vi "AlazarSetTriggerOperation.vi"(0 "Handle":u64, 1 "Trigger Operation":u32(ring) items=["J", "K", "J OR K", "J AND K", "J XOR K", "J AND NOT K", "NOT J AND K"], 5 "error in (no error)":errorcluster, 6 "Trigger Engine 1":u32(ring) items=["J", "K"], 7 "Trigger Engine 2":u32(ring)=1 items=["J", "K"], 8 "Source 1":u32(ring) items=["A", "B", "External", "Disable", "C", "D"], 9 "Source 2":u32(ring)=3 items=["A", "B", "External", "Disable", "C", "D"], 10 "Slope 1":u32(ring)=1 items=["Positive"=1, "Negative"=2], 11 "Slope 2":u32(ring)=1 items=["Positive"=1, "Negative"=2], 12 "Level 1":u32, 13 "Level 2":u32) -> (14 "Handle":u64, 18 "Return Code":u32, 19 "error out":errorcluster)   [LabVIEW 2018]
doc: "Configure the trigger system."
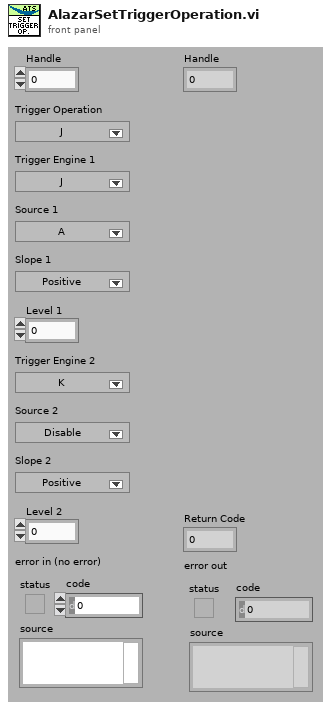
[diagram p1: front panel]
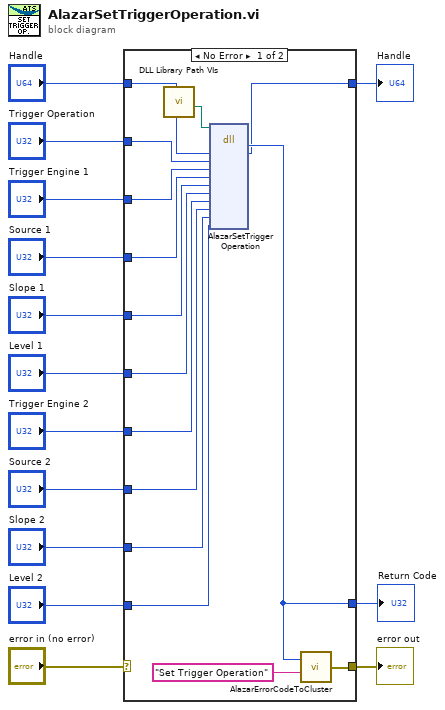
[diagram p0: block diagram]
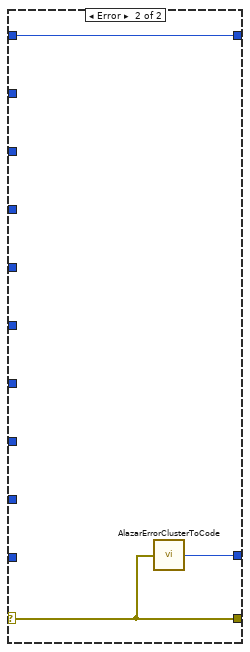
[diagram p2: hidden frame]
diagram:
  n1 = case shown="No Error" "error in (no error)" {
    selector: "error in (no error)" -> [_ w32]
    tunnel: [w26 w32] -> w13
    tunnel: [w28 w31] -> w12
    tunnel: "Handle" -> [w29 w30]
    tunnel: [w25 w30] -> w10
    tunnel: "Trigger Operation" -> [w24 _]
    tunnel: "Trigger Engine 1" -> [w23 _]
    tunnel: "Source 1" -> [w22 _]
    tunnel: "Slope 1" -> [w21 _]
    tunnel: "Level 1" -> [w20 _]
    tunnel: "Trigger Engine 2" -> [w19 _]
    tunnel: "Source 2" -> [w18 _]
    tunnel: "Slope 2" -> [w17 _]
    tunnel: "Level 2" -> [w16 _]
    frame No Error {
      n2 = call "DLL Library Path VIs.vi"() -> ("Alazar"=w15:path)  [unwired: 6 in, 5 out]
      n3 = dll-call lib="C:/Project/SerialSectOCT - FFT GPU/SerialSectOCT/Labview Software/DLL/ATSApi.dll" fn="AlazarSetTriggerOperation"(path in=w15, "handle"=w29, "triggerOperation"=w24, "triggerEngine1"=w23, "source1"=w22, "slope1"=w21, "level1"=w20, "triggerEngine2"=w19, "source2"=w18, "slope2"=w17, "level2"=w16) -> ("return type"=w28:u32, "handle"=w25:u64)  [unwired: 11 in, 2 out]
      n4 = call "AlazarErrorCodeToCluster.vi"("Message"="Set Trigger Operation", "Error Code"=w28) -> ("error out"=w26:errorcluster)
    }
    frame Error {
      n5 = call "AlazarErrorClusterToCode.vi"("error in (no error)"=w32) -> ("Error Code"=w31:u32)
    }
  }
  "Handle" <- w10
  "error out" <- w13
  "Return Code" <- w12
